vi "New Thread Parameters Error.vi"(7 "error source vi name":string, 11 "error":T1) -> (1 "new offset":i32, 3 "error out":errorcluster)   [LabVIEW 2017, in "DSF Core.lvlib" / "Thread Parameters.lvclass"]
uses:
  Thread Parameters.lvclass
  Errors.ctl
  Shared/Constants/Engine Library Name.vi
  <vilib>/NI/Memory Manager/VIs/New Error Cluster Constant (512B).vi
  <vilib>/NI/Memory Manager/Static Error Handling.lvlib
  DSF Core.lvlib
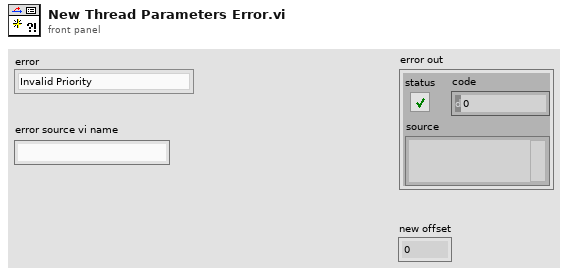
[diagram p1: front panel]
types:
  T1 = typedef "DSF Core.lvlib/Thread Parameters.lvclass/Errors.ctl" = enum16{"Invalid Priority", "Invalid ID"}
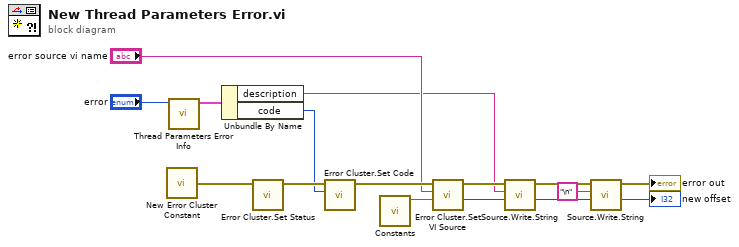
[diagram p0: block diagram]
diagram:
  n1 = call-poly <vilib>:"New Error Cluster Constant.vi"() -> ("error out"=w15:errorcluster)  [unwired: 1 in]
  n2 = call "Thread Parameters Error Info.vi"("error"="error") -> ("error info"=w13:cluster{"code":i32, "description":string})  [unwired: 10 in]
  n3 = Unbundle By Name(w13) -> ("description"=w6:string, "code"=w12:i32)
  n4 = call <vilib>:"Error Cluster.Set Status.vi"("error in"=w15) -> ("error out"=w14:errorcluster)  [unwired: 10 in]
  n5 = call <vilib>:"Error Cluster.Set Code.vi"("code"=w12, "error in"=w14) -> ("error out"=w11:errorcluster)  [unwired: 9 in]
  n6 = call-poly "Constants.vi"() -> ("Engine Library Name"=w9:string)  [unwired: 11 in]
  n7 = call <vilib>:"Error Cluster.Set VI Source.vi"("library name (\"\")"=w9, "vi name"="error source vi name", "error in"=w11) -> ("new offset"=w7:i32, "error out"=w8:errorcluster)  [unwired: 7 in]
  n8 = call <vilib>:"Source.Write.String.vi"("offset"=w7, "string"=w6, "error in"=w8) -> ("new offset"=w3:i32, "error out"=w5:errorcluster)  [unwired: 7 in]
  n9 = call <vilib>:"Source.Write.String.vi"("offset"=w3, "string"="\n", "error in"=w5) -> ("new offset"=→"new offset":i32, "error out"=→"error out":errorcluster)  [unwired: 7 in]
